vi "Write Communication .vi"(8 "error in (no error)":errorcluster, 10 "Communication":T1, 11 "RoomAlert in":refnum<class "RoomAlert.lvclass">) -> (0 "error out":errorcluster, 3 "RoomAlert out":refnum<class "RoomAlert.lvclass">)   [LabVIEW 2018, in "SensorPlugins.lvlib" / "RoomAlert.lvclass"]
uses:
  RoomAlert.lvclass
  TypeDefinitions/CommunicationControls.ctl
  RoomAlert.lvclass/RoomAlert.ctl
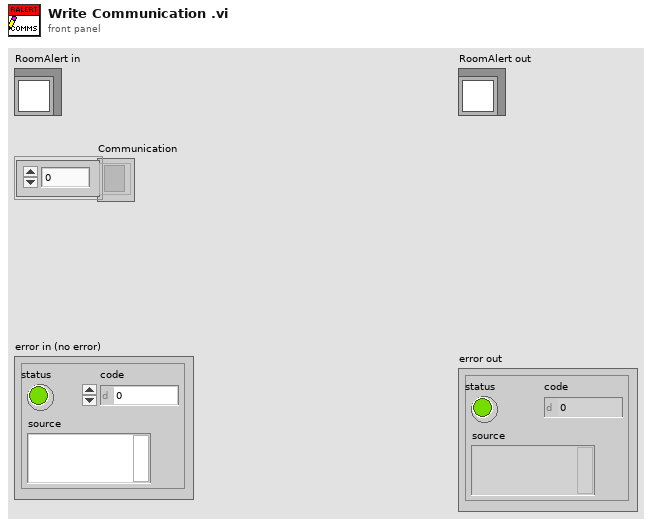
[diagram p1: front panel]
types:
  T1 = typedef "SensorPlugins.lvlib/RoomAlert.lvclass/CommunicationControls.ctl" = refnum<k16>[]
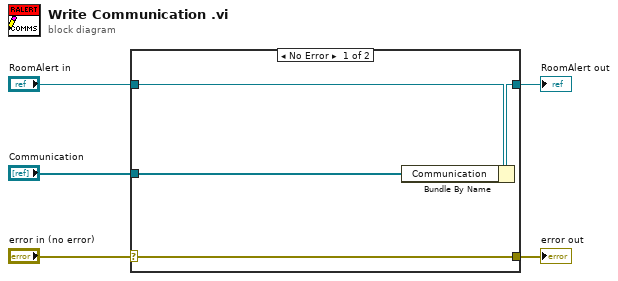
[diagram p0: block diagram]
diagram:
  n1 = case shown="No Error" "error in (no error)" {
    selector: "error in (no error)" -> [w9 w10]
    tunnel: [w9 w10] -> w4
    tunnel: [w7 w11] -> w2
    tunnel: "RoomAlert in" -> [w8 w11]
    tunnel: "Communication" -> [w6 _]
    frame No Error {
      n2 = Bundle By Name(cluster=w8, "Communication"=w6) -> (w7:refnum<class "RoomAlert.lvclass">)
    }
    frame Error {
    }
  }
  "error out" <- w4
  "RoomAlert out" <- w2
